vi "AFGTest.vi"() -> ()   [LabVIEW 2019]
uses:
  AFG3022B_class/AFG3022B.lvclass
panel:
  in  "VISA resource name":refnum<visa-resource-name>
  in  "Channel (0: Channel 1)":u16(ring) items=["Channel 1", "Channel2"]
  in  "Enable Output (T: Enable)":bool=TRUE
  in  "ConfigData":T1={"Frequency (1000 Hz)"=1000.0, "Channel (0: Channel 1)"=0, "Waveform Function (0: Sine)"=0, "Amplitude (1 Vpp)"=1.0, "DC Offset (0.00 V)"=0.0, "Phase Level (-1)"=-1.0, "Phase Unit (0: Radian)"=0} {"Phase Unit (0: Radian)" items=["Radians", "Degrees"]; "Waveform Function (0: Sine)" items=["Sine", "Square", "Pulse", "Ramp", "Noise", "DC", "Sin(x)/x", "Gaussian", "Lorentz", "Exponential Rise", "Exponential Decay", "Haversine"]; "Channel (0: Channel 1)" items=["Channel 1", "Channel 2"]}
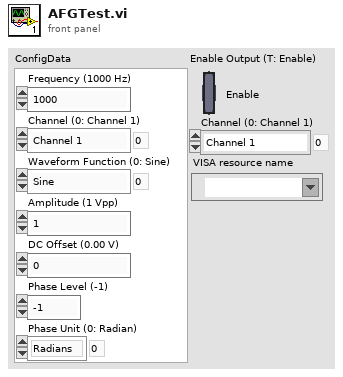
[diagram p1: front panel]
types:
  T1 = cluster{"Frequency (1000 Hz)":dbl, "Channel (0: Channel 1)":u16, "Waveform Function (0: Sine)":u16, "Amplitude (1 Vpp)":dbl, "DC Offset (0.00 V)":dbl, "Phase Level (-1)":dbl, "Phase Unit (0: Radian)":u16}
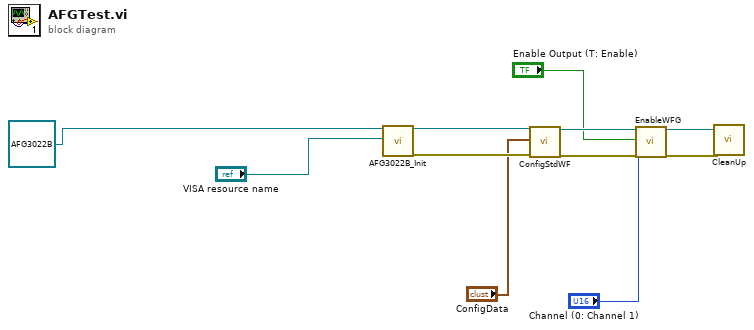
[diagram p0: block diagram]
diagram:
  n1 = call "AFG3022B_Init.vi"("object in"=refnum<class "AFG3022B.lvclass"> refnum ("AFG3022B"), "VISA resource name"="VISA resource name") -> ("object out"=w10:refnum<class "AFG3022B.lvclass">, "error out"=w8:errorcluster)  [unwired: 16 in]
  n2 = call-dynamic "ConfigStdWF.vi"("object in"=w10, "ConfigData"="ConfigData", "error in (no error)"=w8) -> ("object out"=w9:refnum<class "AFG3022B.lvclass">, "error out"=w7:errorcluster)  [unwired: 15 in]
  n3 = call-dynamic "EnableWFG.vi"("object in"=w9, "Enable Output (T: Enable)"="Enable Output (T: Enable)", "Channel (0: Channel 1)"="Channel (0: Channel 1)", "error in (no error)"=w7) -> ("object out"=w3:refnum<class "AFG3022B.lvclass">, "error out"=w2:errorcluster)  [unwired: 14 in]
  n4 = call-dynamic "CleanUp.vi"("object in"=w3, "error in (no error)"=w2) -> ()  [unwired: 16 in, 2 out]
